vi "Offsets.vi"(8 "error in (no error)":errorcluster, 9 "Dataset Trans Id":T1, 10 "Data In":dbl[](array[numeric]), 11 "DAO Actions":T5) -> (0 "error out":errorcluster, 2 "Data Out":dbl[](array[numeric]), 4 "Labels":string[](array[string]))   [LabVIEW 2009]
uses:
  Data Access Objects/Metadata/DAO Actions with Remove.ctl
  Global Data/Dataset Transaction Id.ctl
  Global Data/Dataset Source.ctl
  Global Data/Dataset Type.ctl
  Apps/Yes No Button.ctl
panel:
  out "Offsets":variant
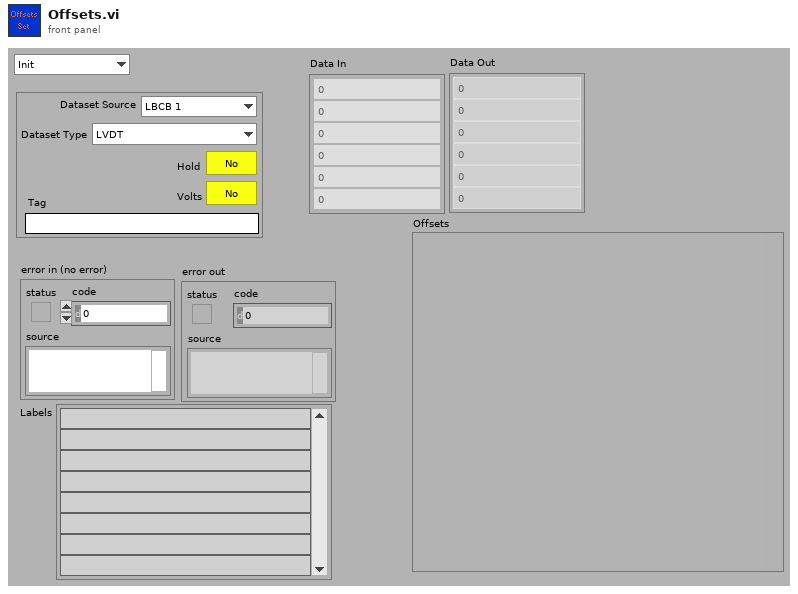
[diagram p1: front panel]
types:
  T1 = typedef "Dataset Transaction Id.ctl" = cluster{"Dataset Source":T2, "Dataset Type":T3, "Hold":T4, "Volts":T4, "Tag":string}
  T2 = typedef "Dataset Source.ctl" = enum16{"LBCB 1", "LBCB 2", "Combined", "External Sensors"}
  T3 = typedef "Dataset Type.ctl" = enum16{"LVDT", "Load Cell", "Actuator Command", "Servo Error", "Displacement Command", "Displacement", "Force"}
  T4 = typedef "Yes No Button.ctl" = bool
  T5 = typedef "DAO Actions with Remove.ctl" = enum16{"Init", "Get", "Set", "Remove"}
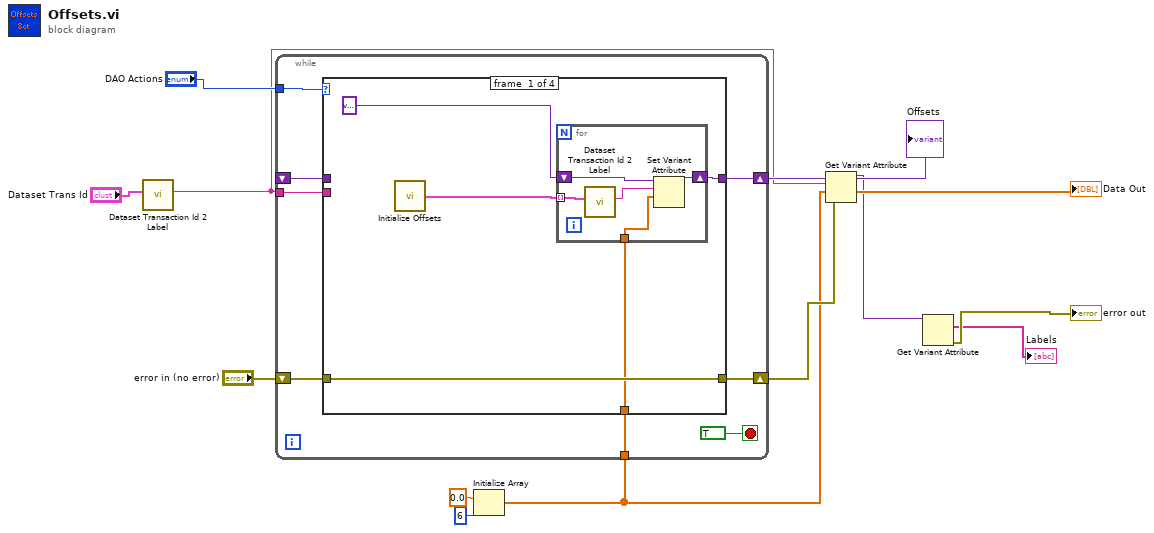
[diagram p0: block diagram]
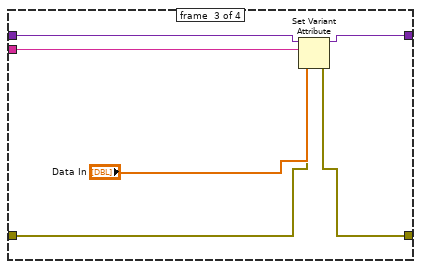
[diagram p3: hidden frame]
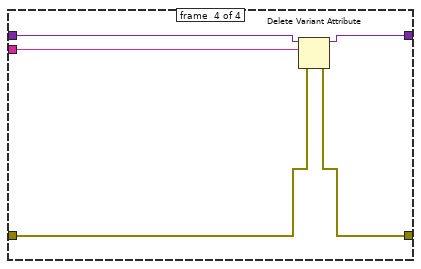
[diagram p4: hidden frame]
diagram:
  n1 = call "Dataset Transaction Id 2 Label.vi"("Dataset Trans Id"="Dataset Trans Id") -> ("Label"=w6:string)  [unwired: 10 in]
  n2 = Initialize Array(0.0 ("element"), 6 ("dimension size")) -> (w1:dbl[])
  n3 = while {
    tunnel: "DAO Actions" -> [w20]
    tunnel: w6 -> [w19]
    shift-right: [w17] -> w8
    shift-left: _ -> [w18]
    shift-right: [w15] -> w7
    shift-left: "error in (no error)" -> [w16]
    tunnel: w1 -> [w14]
    stop <- TRUE stop-if-true
    n4 = case shown="\"Set\"" w20 {
      tunnel: w19 -> [_ _ w38 w44]
      tunnel: w18 -> [_ w33 w37 w43]
      tunnel: [w24 w33 w36 w42] -> w17
      tunnel: w16 -> [w26 w32 w35 w41]
      tunnel: [w26 w32 w34 w40] -> w15
      tunnel: w14 -> [w23 _ _ _]
      frame #0 {
        n5 = call "Initialize Offsets.vi"() -> ("Transactions"=w22:T1[])
        n6 = for {
          tunnel: w23 -> [w28]
          tunnel: w22 -> [w27] mode=indexing
          shift-right: [w30] -> w24
          shift-left: variant -> [w31]
          n7 = call "Dataset Transaction Id 2 Label.vi"("Dataset Trans Id"=w27) -> ("Label"=w29:string)  [unwired: 10 in]
          n8 = Set Variant Attribute(Variant=w31, name=w29, value=w28) -> (Variant out=w30:variant)  [unwired: 1 in, 2 out]
        }
      }
      frame #1 {
      }
      frame #2 {
        n9 = Set Variant Attribute(Variant=w37, name=w38, value="Data In", error in=w35) -> (Variant out=w36:variant, error out=w34:errorcluster)  [unwired: 1 out]
      }
      frame #3 {
        n10 = Delete Variant Attribute(4:w41, 6:w44, 7:w43) -> (0:w40:errorcluster, 3:w42:variant)  [unwired: 1 out]
      }
    }
  }
  "Offsets" <- w8
  n11 = Get Variant Attribute(Variant=w8, name=w6, default value (empty Variant)=w1, error in=w7) -> (duplicate Variant=w4:variant, value=→"Data Out":dbl[])  [unwired: 2 out]
  n12 = Get Variant Attribute(Variant=w4) -> (names=→"Labels":string[], error out=→"error out":errorcluster)  [unwired: 3 in, 2 out]
